vi "Lab1_2_feedback.vi"() -> ()   [LabVIEW 2020]
panel:
  in  "Add number":bool
  out "Number Being Added":i32
  out "Array":i32[](array[numeric])
  in  "stop":bool
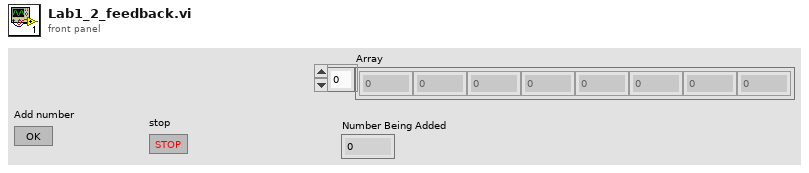
[diagram p1: front panel]
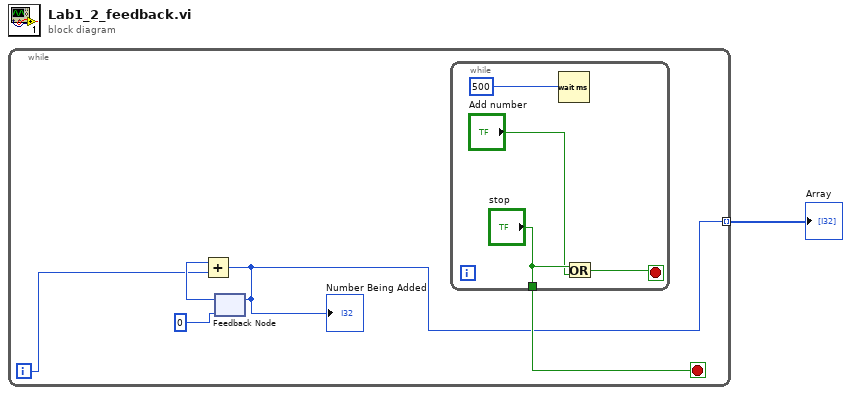
[diagram p0: block diagram]
diagram:
  n1 = while {
    tunnel: [w3] -> w1 mode=indexing
    i -> [w2]
    stop <- w6 stop-if-true
    n2 = feedback #1(0) -> (w5:i32)
    n3 = Add(x=w5, y=w2) -> (x+y=w3:i32)
    "Number Being Added" <- w3
    n4 = feedback-in #1(w3) -> ()
    n5 = while {
      tunnel: ["stop"] -> w6
      stop <- w8 stop-if-true
      n6 = Wait (ms)(milliseconds to wait=u32 500) -> ()  [unwired: 1 out]
      n7 = Or(x="stop", y="Add number") -> (x .or. y?=w8:bool)
    }
  }
  "Array" <- w1
